vi "ACK_To_Data.vi"(6 "LogiPul":i32, 8 "MaxCH":i32, 10 "Size":T2, 11 "String":string) -> (2 "Bin_Data_All":i32[][](array[numeric]), 3 "Bin Data":T1)   [LabVIEW 2017]
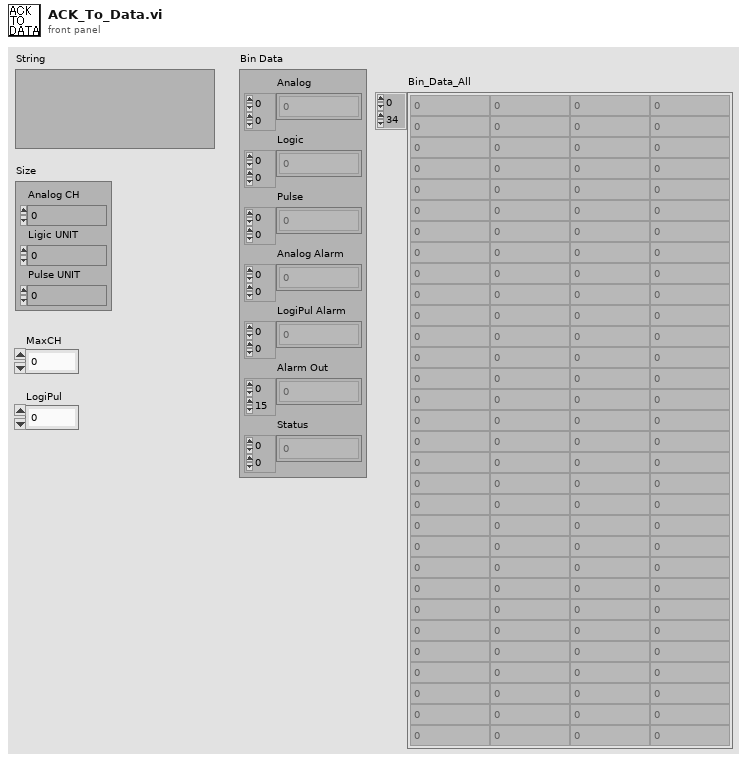
[diagram p1: front panel]
types:
  T1 = cluster{"Analog":i16[][], "Logic":u8[][], "Pulse":i32[][], "Analog Alarm":u8[][], "LogiPul Alarm":u8[][], "Alarm Out":u8[][], "Status":u8[][]}
  T2 = cluster{"Analog CH":i32, "Ligic UNIT":i32, "Pulse UNIT":i32}
  T3 = cluster{i16[][], "Bit[]":u8[][], i32[][], "Bit[]":u8[][], "Bit[]":u8[][], "Bit[]":u8[][], "Bit[]":u8[][]}
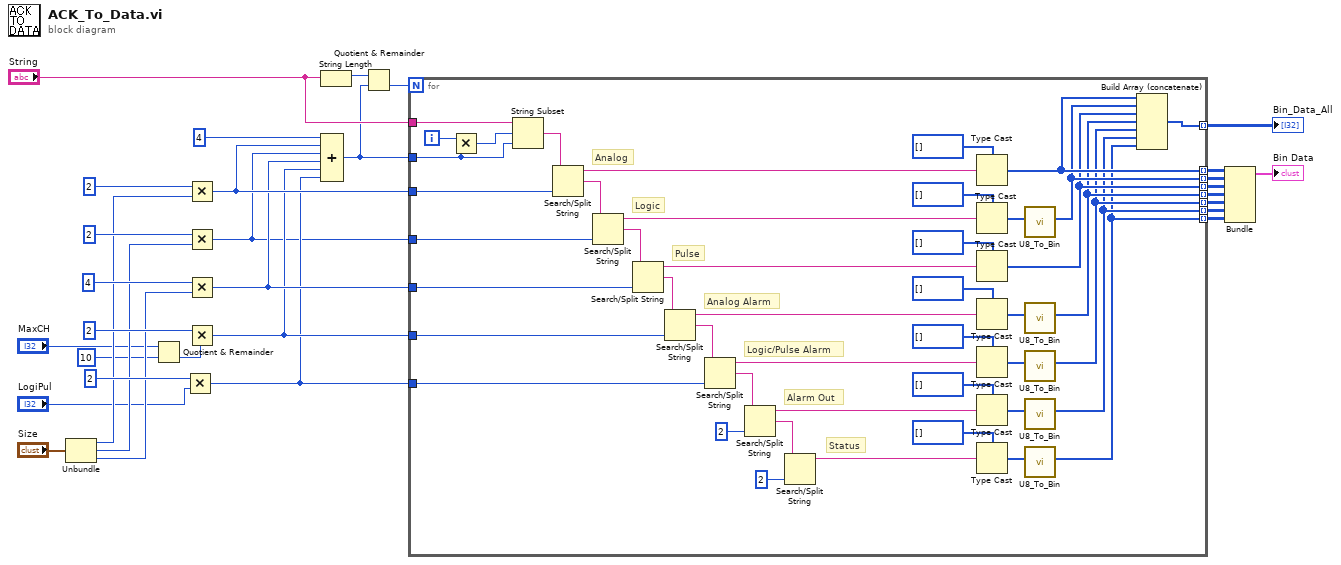
[diagram p0: block diagram]
diagram:
  n1 = Unbundle("Size") -> ("Analog CH"=w16:i32, "Ligic UNIT"=w15:i32, "Pulse UNIT"=w14:i32)
  n2 = Quotient & Remainder(x="MaxCH", y=10) -> (floor(x/y)=w13:i32)  [unwired: 1 out]
  n3 = Multiply(x=2 ("y"), y="LogiPul") -> (x*y=w21:i32)
  n4 = Multiply(x=2 ("y"), y=w16) -> (x*y=w29:i32)
  n5 = Multiply(x=2 ("y"), y=w15) -> (x*y=w18:i32)
  n6 = Multiply(x=4 ("y"), y=w14) -> (x*y=w28:i32)
  n7 = Multiply(x=2 ("y"), y=w13) -> (x*y=w22:i32)
  n8 = String Length(string="String") -> (length=w26:i32)
  n9 = Compound Arithmetic op=ADD(4 ("value"), w29, w18, w28, w22, w21) -> (w23:i32)
  n10 = Quotient & Remainder(x=w26, y=w23) -> (floor(x/y)=w25:i32)  [unwired: 1 out]
  n11 = for {
    N: w25 -> [_]
    tunnel: w29 -> [w51]
    tunnel: w18 -> [w50]
    tunnel: w28 -> [w49]
    tunnel: w22 -> [w48]
    tunnel: w21 -> [w47]
    tunnel: "String" -> [w43]
    tunnel: w23 -> [w45]
    tunnel: [w40] -> w11 mode=indexing
    tunnel: [w39] -> w10 mode=indexing
    tunnel: [w38] -> w9 mode=indexing
    tunnel: [w37] -> w8 mode=indexing
    tunnel: [w36] -> w7 mode=indexing
    tunnel: [w35] -> w6 mode=indexing
    tunnel: [w34] -> w5 mode=indexing
    tunnel: [w33] -> w3 mode=indexing
    i -> [w44]
    # "Status"
    # "Alarm Out"
    # "Logic/Pulse Alarm"
    # "Analog Alarm"
    # "Pulse"
    # "Logic"
    # "Analog"
    n12 = Multiply(x=w44, y=w45) -> (x*y=w46:i32)
    n13 = String Subset(string=w43, offset (0)=w46, length (rest)=w45) -> (substring=w42:string)
    n14 = Search/Split String(string=w42, offset (0)=w51) -> (substring before match=w77:string, match + rest of string=w76:string)  [unwired: 1 in, 1 out]
    n15 = Search/Split String(string=w76, offset (0)=w50) -> (substring before match=w75:string, match + rest of string=w74:string)  [unwired: 1 in, 1 out]
    n16 = Search/Split String(string=w74, offset (0)=w49) -> (substring before match=w73:string, match + rest of string=w72:string)  [unwired: 1 in, 1 out]
    n17 = Search/Split String(string=w72, offset (0)=w48) -> (substring before match=w71:string, match + rest of string=w68:string)  [unwired: 1 in, 1 out]
    n18 = Search/Split String(string=w68, offset (0)=w47) -> (substring before match=w70:string, match + rest of string=w67:string)  [unwired: 1 in, 1 out]
    n19 = Search/Split String(string=w67, offset (0)=2) -> (substring before match=w69:string, match + rest of string=w65:string)  [unwired: 1 in, 1 out]
    n20 = Search/Split String(string=w65, offset (0)=2) -> (substring before match=w64:string)  [unwired: 1 in, 2 out]
    n21 = Type Cast(type=i16[] [], x=w77) -> (*(type *) &x=w40:i16[])
    n22 = Type Cast(type=u16[] [], x=w75) -> (*(type *) &x=w41:u16[])
    n23 = Type Cast(type=i32[] [], x=w73) -> (*(type *) &x=w38:i32[])
    n24 = Type Cast(type=u16[] [], x=w71) -> (*(type *) &x=w53:u16[])
    n25 = Type Cast(type=u16[] [], x=w70) -> (*(type *) &x=w52:u16[])
    n26 = Type Cast(type=u16[] [], x=w69) -> (*(type *) &x=w55:u16[])
    n27 = Type Cast(type=u16[] [], x=w64) -> (*(type *) &x=w54:u16[])
    n28 = call "U8_To_Bin.vi"("U16[]"=w41) -> ("Bit[]"=w39:u8[])  [unwired: 10 out]
    n29 = call "U8_To_Bin.vi"("U16[]"=w53) -> ("Bit[]"=w37:u8[])  [unwired: 10 out]
    n30 = call "U8_To_Bin.vi"("U16[]"=w52) -> ("Bit[]"=w36:u8[])  [unwired: 10 out]
    n31 = call "U8_To_Bin.vi"("U16[]"=w55) -> ("Bit[]"=w35:u8[])  [unwired: 10 out]
    n32 = call "U8_To_Bin.vi"("U16[]"=w54) -> ("Bit[]"=w34:u8[])  [unwired: 10 out]
    n33 = Build Array (concatenate)(w40, w39, w38, w37, w36, w35, w34) -> (w33:i32[])
  }
  "Bin_Data_All" <- w3
  n34 = Bundle(w11, "Bit[]"=w10, w9, "Bit[]"=w8, "Bit[]"=w7, "Bit[]"=w6, "Bit[]"=w5) -> (→"Bin Data":T3)  [unwired: 1 out]
